vi "Read Error.vi"(8 "error in (no error)":errorcluster, 11 "MySQL initial erroe in":refnum<class "MySQL initial error.lvclass">) -> (0 "error out":errorcluster, 2 "Error":bool, 3 "MySQL initial erroe out":refnum<class "MySQL initial error.lvclass">)   [LabVIEW 2019, in "DataBase.lvlib" / "MySQL initial error.lvclass"]
uses:
  MySQL initial error.lvclass
  MySQL initial error.lvclass/MySQL initial error.ctl
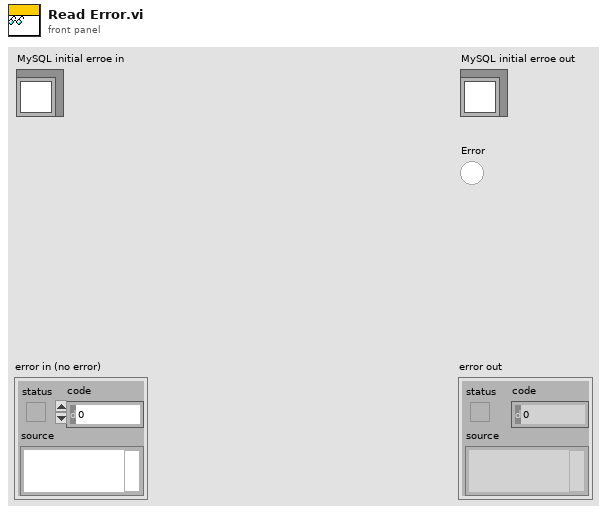
[diagram p1: front panel]
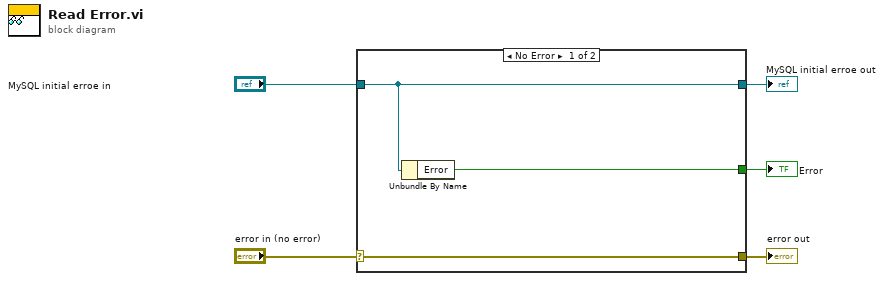
[diagram p0: block diagram]
diagram:
  n1 = case shown="No Error" "error in (no error)" {
    selector: "error in (no error)" -> [w8 w9]
    tunnel: [w8 w9] -> w4
    tunnel: [w7 w10] -> w2
    tunnel: "MySQL initial erroe in" -> [w7 w10]
    tunnel: [w6 _] -> w1
    frame No Error {
      n2 = Unbundle By Name(w7) -> ("Error"=w6:bool)
    }
    frame Error {
    }
  }
  "error out" <- w4
  "MySQL initial erroe out" <- w2
  "Error" <- w1
